vi "Untitled 6.vi"() -> ()   [LabVIEW 2017]
uses:
  Global 1.vi
panel:
  in  "stop 2":bool
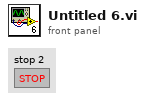
[diagram p1: front panel]
types:
  T1 = enum16{"Standard", "Buffered", "CRLF", "Immediate"}
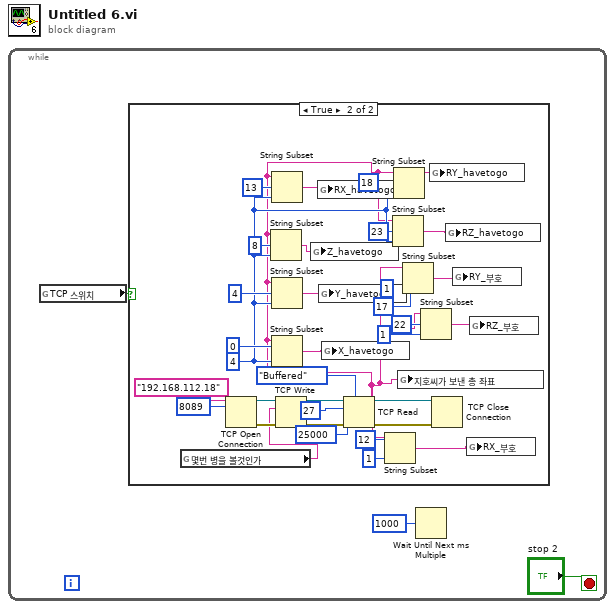
[diagram p0: block diagram]
diagram:
  n1 = while {
    stop <- "stop 2" stop-if-true
    n2 = global read "Global 1.vi" "TCP 스위치"() -> (w2:bool)
    n3 = case shown="True" w2 {
      frame False {
      }
      frame True {
        w32 = 4 ("length (rest)")
        n4 = global read "Global 1.vi" "몇번 병을 볼것인가"() -> (w23:string)
        n5 = TCP Open Connection(address="192.168.112.18", remote port or service name=u16 8089) -> (connection ID=w27:refnum<k5>, error out=w26:errorcluster)  [unwired: 3 in]
        n6 = TCP Write(connection ID=w27, data in=w23, error in (no error)=w26) -> (connection ID out=w25:refnum<k5>, error out=w24:errorcluster)  [unwired: 1 in, 1 out]
        n7 = TCP Read(connection ID=w25, bytes to read=27, error in (no error)=w24, 7:T1."Buffered" ("mode (standard)"), 9:25000 ("timeout ms (25000)")) -> (connection ID out=w36:refnum<k5>, data out=w10:string, error out=w35:errorcluster)
        n8 = String Subset(string=w10, offset (0)=8, length (rest)=w32) -> (substring=w14:string)
        n9 = String Subset(string=w10, offset (0)=13, length (rest)=w32) -> (substring=w13:string)
        n10 = String Subset(string=w10, offset (0)=4, length (rest)=w32) -> (substring=w15:string)
        n11 = String Subset(string=w10, offset (0)=0, length (rest)=w32) -> (substring=w16:string)
        n12 = global write "Global 1.vi" "Z_havetogo"(w14) -> ()
        n13 = global write "Global 1.vi" "RX_havetogo"(w13) -> ()
        n14 = global write "Global 1.vi" "Y_havetogo"(w15) -> ()
        n15 = global write "Global 1.vi" "X_havetogo"(w16) -> ()
        n16 = String Subset(string=w10, offset (0)=12, length (rest)=1 ("length (rest)")) -> (substring=w9:string)
        n17 = String Subset(string=w10, offset (0)=23, length (rest)=w32) -> (substring=w11:string)
        n18 = String Subset(string=w10, offset (0)=18, length (rest)=w32) -> (substring=w12:string)
        n19 = global write "Global 1.vi" "지호씨가 보낸 총 좌표"(w10) -> ()
        n20 = String Subset(string=w10, offset (0)=17, length (rest)=1 ("length (rest)")) -> (substring=w8:string)
        n21 = String Subset(string=w10, offset (0)=22, length (rest)=1 ("length (rest)")) -> (substring=w7:string)
        n22 = global write "Global 1.vi" "RY_havetogo"(w12) -> ()
        n23 = TCP Close Connection(connection ID=w36, error in (no error)=w35) -> ()  [unwired: 1 in, 2 out]
        n24 = global write "Global 1.vi" "RZ_havetogo"(w11) -> ()
        n25 = global write "Global 1.vi" "RY_부호"(w8) -> ()
        n26 = global write "Global 1.vi" "RX_부호"(w9) -> ()
        n27 = global write "Global 1.vi" "RZ_부호"(w7) -> ()
      }
    }
    n28 = Wait Until Next ms Multiple(millisecond multiple=u32 1000) -> ()  [unwired: 1 out]
  }
